vi "Data.vi"(11 "Message Queues out":T1) -> ()   [LabVIEW 2024]
doc: "This vi used for Data Logging Loop and its process"
uses:
  Message Queue/All Message Queues.ctl
  Message Queue/Message Cluster.ctl
  controls/GlobalData.ctl
  Message Queue/Enqueue Message (Single).vi
  <vilib>/Utility/error.llb/Error Cluster From Error Code.vi
  <vilib>/ErrorRing/Error Ring.xnode
  Message Queue/Message Queue.lvlib
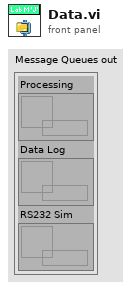
[diagram p1: front panel]
types:
  T1 = typedef "Message Queue.lvlib/All Message Queues.ctl" = cluster{"Processing":refnum<queue>, "Data Log":refnum<queue>, "RS232 Sim":refnum<queue>}
  T2 = typedef "GlobalData.ctl" = cluster{"Measurements":cluster{"Measurement Graphs":refnum<vi>, "Pressure":refnum<vi>, "Temperature":refnum<vi>, "Salinity":refnum<vi>, "Weight":refnum<vi>, "Pressure Raw":refnum<vi>, "Temperature Raw":refnum<vi>, "Salinity Raw":refnum<vi>, "Weight Raw":refnum<vi>, "Measurement Statstics":refnum<vi>, "Time Array":refnum<vi>}, "Settings":cluster{"Sampling Settings":refnum<vi>, "General Settings":refnum<vi>, "Disable Sensor Reading":refnum<vi>, "Units Settings":refnum<vi>, "Channels Settings":refnum<vi>, "Weight Port Settings":refnum<vi>}, "Calibration Data":cluster{"Pressure Cal":refnum<vi>, "Temperature Cal":refnum<vi>, "Salinity Cal":refnum<vi>, "Weight Cal":refnum<vi>}, "UI":cluster{"Generate Report":refnum<vi>}}
  T3 = enum16{"open", "open or create", "create or replace", "create", "open (read-only)"}
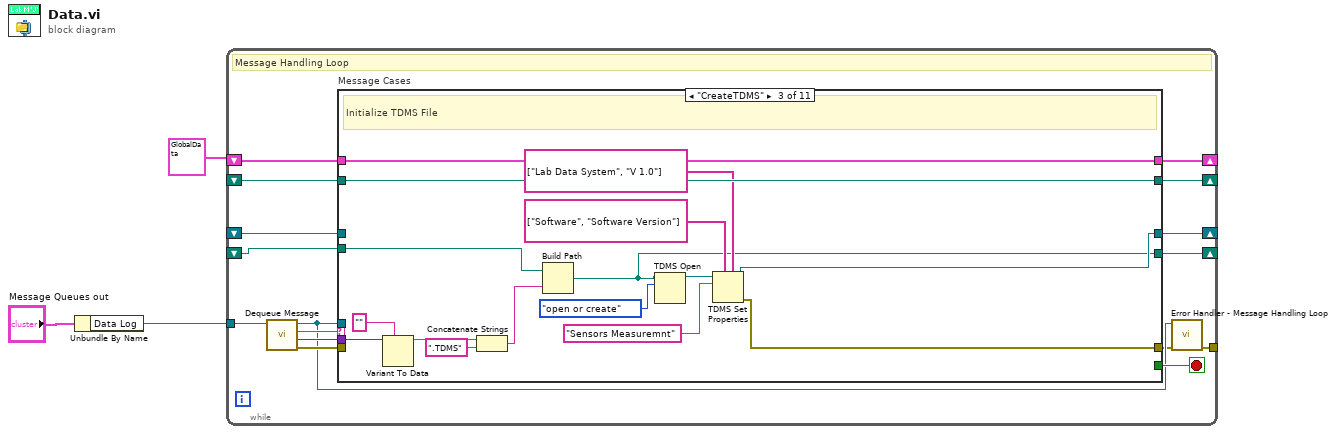
[diagram p0: block diagram]
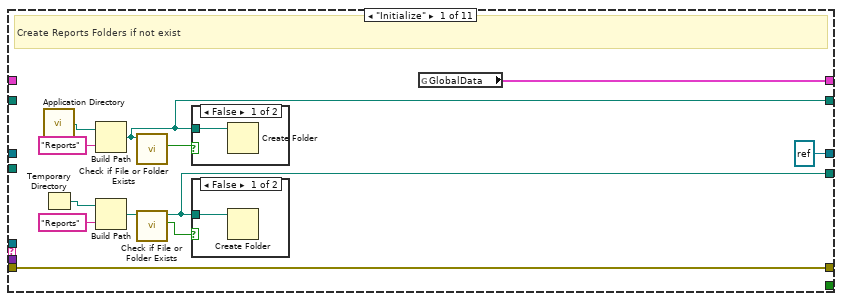
[diagram p2: hidden frame]
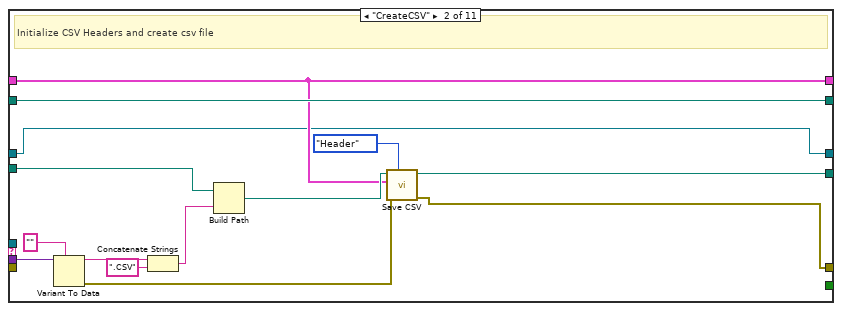
[diagram p5: hidden frame]
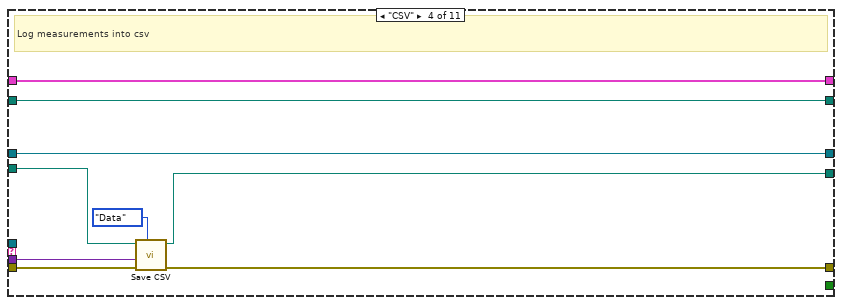
[diagram p6: hidden frame]
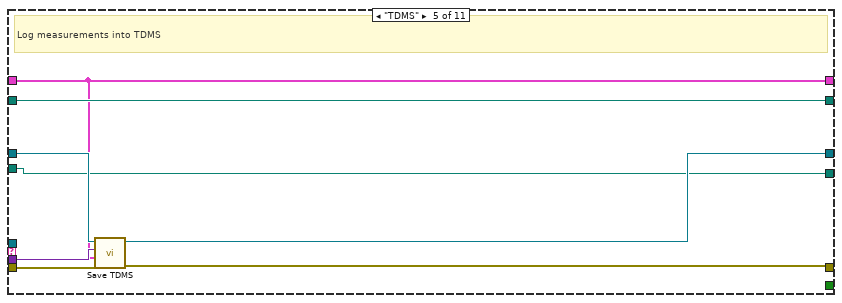
[diagram p7: hidden frame]
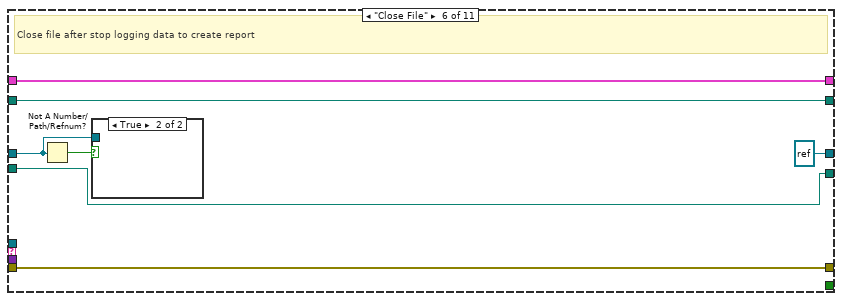
[diagram p8: hidden frame]
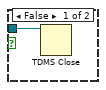
[diagram p9: hidden frame]
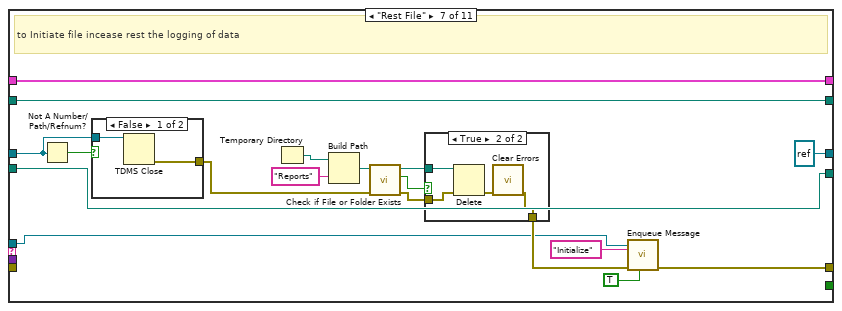
[diagram p10: hidden frame]
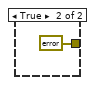
[diagram p12: hidden frame]
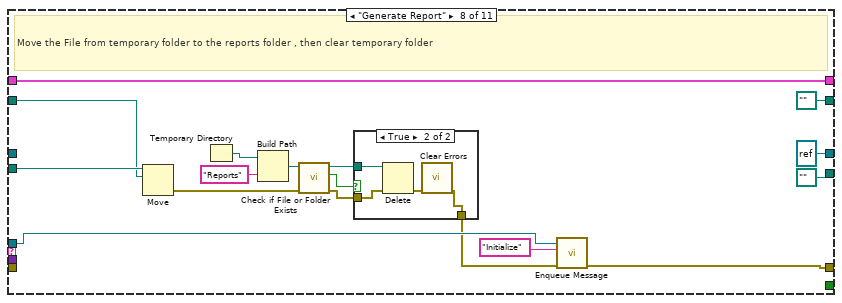
[diagram p13: hidden frame]
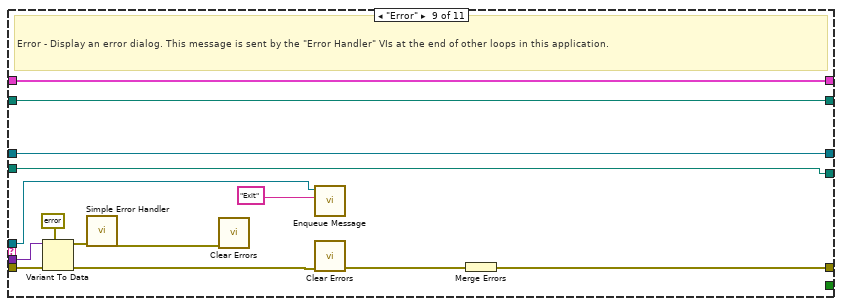
[diagram p15: hidden frame]
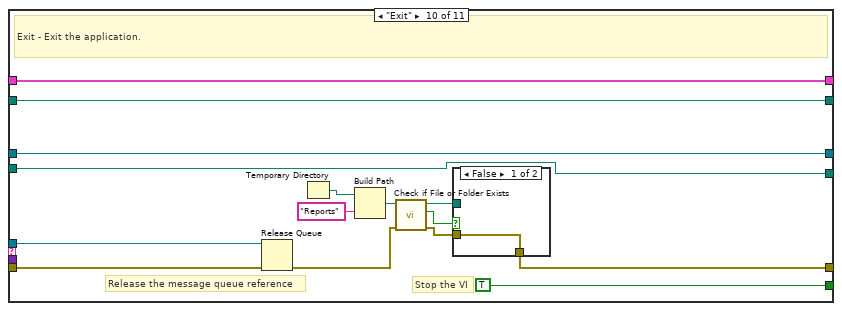
[diagram p16: hidden frame]
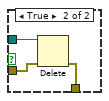
[diagram p17: hidden frame]
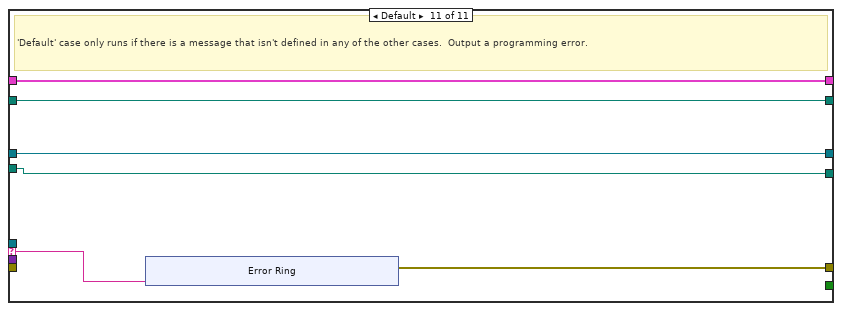
[diagram p18: hidden frame]
diagram:
  n1 = Unbundle By Name("Message Queues out") -> ("Data Log"=w3:refnum<queue>)
  n2 = while {
    shift-right: [w18] -> _
    shift-left: T2 {"Measurements"={"Measurement Graphs"=refnum, "Pressure"=refnum, "Temperature"=refnum, "Salinity"=refnum, "Weight"=refnum, "Pressure Raw"=refnum, "Temperature Raw"=refnum, "Salinity Raw"=refnum, "Weight Raw"=refnum, "Measurement Statstics"=refnum, "Time Array"=refnum}, "Settings"={"Sampling Settings"=refnum, "General Settings"=refnum, "Disable Sensor Reading"=refnum, "Units Settings"=refnum, "Channels Settings"=refnum, "Weight Port Settings"=refnum}, "Calibration Data"={"Pressure Cal"=refnum, "Temperature Cal"=refnum, "Salinity Cal"=refnum, "Weight Cal"=refnum}, "UI"={"Generate Report"=refnum}} ("GlobalData") -> [w19]
    tunnel: w3 -> [w4]
    tunnel: [w12] -> _
    shift-right: [w10] -> _
    shift-left: _ -> [w7]
    shift-right: [w9] -> _
    shift-left: _ -> [w8]
    shift-right: [w6] -> _
    shift-left: _ -> [w5]
    stop <- w17 stop-if-true
    # "Message Handling Loop"
    n3 = call "Dequeue Message.vi"("Message Queue"=w4) -> ("error out"=w16:errorcluster, "Message Data"=w14:variant, "Message"=w15:string, "dup Message Queue"=w13:refnum<queue>)  [unwired: 7 in]
    n4 = case "Message Cases" shown="\"CreateTDMS\"" w15 {
      selector: w15 -> [_ _ _ _ _ _ _ _ _ _ w173]
      tunnel: w13 -> [_ _ _ _ _ _ w91 w126 w137 w165 _]
      tunnel: w16 -> [w31 _ _ w69 w79 w87 _ _ w150 w162 _]
      tunnel: [w31 w35 w48 w66 w78 w87 w92 w127 w145 w155 w174] -> w11
      tunnel: w19 -> [_ w37 w63 w72 w73 w86 w106 w131 w149 w164 w175]
      tunnel: [w30 w37 w63 w72 w73 w86 w106 w131 w149 w164 w175] -> w18
      tunnel: [_ _ _ _ _ _ _ _ _ TRUE _] -> w17
      tunnel: w14 -> [_ w47 w62 w68 w76 _ _ _ w148 _ _]
      tunnel: [w22 w42 w56 w71 w74 w83 w103 path "" ("appended path") w144 w153 w170] -> w10
      tunnel: [w21 w40 w49 w65 w75 w81 w101 path "" ("new file path (Not A Path if cancelled)") w142 w151 w172] -> w9
      tunnel: w8 -> [_ w41 w57 w67 w75 w81 w101 w130 w142 w151 w172]
      tunnel: w7 -> [_ w42 w56 w71 w74 w83 w103 w129 w144 w153 w170]
      tunnel: [refnum<k34> refnum ("tdms file out") w34 w50 w70 w77 refnum<k34> refnum ("tdms file out") refnum<k34> refnum ("tdms file out") refnum<k34> refnum ("tdms file out") w143 w152 w171] -> w6
      tunnel: w5 -> [_ w34 _ w70 w80 w84 w104 _ w143 w152 w171]
      frame "Initialize" {
        # "Create Reports Folders if not exist"
        n5 = call <vilib>:"Application Directory.vi"() -> ("Application Directory"=w28:path)
        n6 = Temporary Directory() -> (w25:path)
        n7 = Build Path(base path=w28, name or relative path="Reports") -> (appended path=w22:path)
        n8 = Build Path(base path=w25, name or relative path="Reports") -> (appended path=w26:path)
        n9 = call <vilib>:"Check if File or Folder Exists.vi"("path"=w22) -> ("file or folder exists?"=w27:bool)  [unwired: 8 in, 2 out]
        n10 = call <vilib>:"Check if File or Folder Exists.vi"("path"=w26) -> ("file or folder exists?"=w23:bool, "dup path"=w21:path)  [unwired: 8 in, 1 out]
        n11 = case shown="False" w27 {
          tunnel: w22 -> [w33 _]
          frame False {
            n12 = Create Folder(path (use dialog)=w33) -> ()  [unwired: 2 in, 3 out]
          }
          frame True {
          }
        }
        n13 = case shown="False" w23 {
          tunnel: w21 -> [w32 _]
          frame False {
            n14 = Create Folder(path (use dialog)=w32) -> ()  [unwired: 2 in, 3 out]
          }
          frame True {
          }
        }
        n15 = global read "GlobalData.vi" "GlobalData"() -> (w30:T2)
      }
      frame "CreateCSV" {
        # "Initialize CSV Headers and create csv file"
        n16 = Variant To Data(type="", Variant=w47) -> (data=w45:string, error out=w36:errorcluster)  [unwired: 1 in]
        n17 = Concatenate Strings(w45, ".CSV" ("string")) -> (w43:string)
        n18 = Build Path(base path=w41, name or relative path=w43) -> (appended path=w39:path)
        n19 = call "Save CSV.vi"("CSV Type"=enum16{"Header", "Data"}."Header", "error in (no error)"=w36, "GlobalData"=w37, "file path (dialog if empty)"=w39) -> ("error out"=w35:errorcluster, "new file path (Not A Path if cancelled)"=w40:path)  [unwired: 6 in]
      }
      frame "CreateTDMS" {
        # "Initialize TDMS File"
        n20 = Variant To Data(type="", Variant=w62) -> (data=w60:string)  [unwired: 1 in, 1 out]
        n21 = Concatenate Strings(w60, ".TDMS" ("string")) -> (w58:string)
        n22 = Build Path(base path=w57, name or relative path=w58) -> (appended path=w49:path)
        n23 = TDMS Open(10:T3."open or create" ("operation (0:open)"), 11:w49) -> (3:w54:refnum<k34>)  [unwired: 5 in, 1 out]
        n24 = TDMS Set Properties(5:string[] ["Lab Data System", "V 1.0"] ("property names"), 7:string[] ["Software", "Software Version"] ("property names"), 10:"Sensors Measuremnt" ("group name"), 11:w54) -> (0:w48:errorcluster, 3:w50:refnum<k34>)  [unwired: 2 in, 2 out]
      }
      frame "CSV" {
        # "Log measurements into csv"
        n25 = call "Save CSV.vi"("CSV Type"=enum16{"Header", "Data"}."Data", "error in (no error)"=w69, "Data"=w68, "file path (dialog if empty)"=w67) -> ("error out"=w66:errorcluster, "new file path (Not A Path if cancelled)"=w65:path)  [unwired: 6 in]
      }
      frame "TDMS" {
        # "Log measurements into TDMS"
        n26 = call "Save TDMS.vi"("error in (no error)"=w79, "GlobalData"=w73, "Data"=w76, "tdms file in"=w80) -> ("error out"=w78:errorcluster, "tdms file out"=w77:refnum<k34>)  [unwired: 6 in]
      }
      frame "Close File" {
        # "Close file after stop logging data to create report"
        n27 = Not A Number/Path/Refnum?(number/path/refnum=w84) -> (NaN/Path/Refnum?=w85:bool)
        n28 = case shown="True" w85 {
          tunnel: w84 -> [w88 _]
          frame False {
            n29 = TDMS Close(11:w88) -> ()  [unwired: 1 in, 2 out]
          }
          frame True {
          }
        }
      }
      frame "Rest File" {
        # "to Initiate file incease rest the logging of data"
        n30 = Not A Number/Path/Refnum?(number/path/refnum=w104) -> (NaN/Path/Refnum?=w105:bool)
        n31 = case shown="False" w105 {
          tunnel: w104 -> [w113 _]
          tunnel: [w112 errorcluster {"status"=FALSE, "code"=0, "source"=""} ("error out")] -> w90
          frame False {
            n32 = TDMS Close(11:w113) -> (0:w112:errorcluster)  [unwired: 1 in, 1 out]
          }
          frame True {
          }
        }
        n33 = Temporary Directory() -> (w99:path)
        n34 = Build Path(base path=w99, name or relative path="Reports") -> (appended path=w100:path)
        n35 = call <vilib>:"Check if File or Folder Exists.vi"("error in (no error)"=w90, "path"=w100) -> ("error out"=w96:errorcluster, "file or folder exists?"=w98:bool, "dup path"=w97:path)  [unwired: 7 in]
        n36 = case shown="True" w98 {
          tunnel: w97 -> [_ w111]
          tunnel: w96 -> [w107 w110]
          tunnel: [w107 w108] -> w95
          frame False {
          }
          frame True {
            n37 = Delete(path (use dialog)=w111, error in=w110) -> (error out=w109:errorcluster)  [unwired: 3 in, 2 out]
            n38 = call <vilib>:"Clear Errors.vi"("error in (no error)"=w109) -> ("error out"=w108:errorcluster)  [unwired: 5 in, 1 out]
          }
        }
        n39 = call-poly "Enqueue Message.vi"("Priority Message? (F)"=TRUE, "error in (no error)"=w95, "Message"="Initialize", "Message Queue"=w91) -> ("error out"=w92:errorcluster)  [unwired: 6 in, 1 out]
      }
      frame "Generate Report" {
        # "Move the File from temporary folder to the reports folder , then clear temporary folder"
        n40 = Move(source path=w130, 10:w129) -> (error out=w119:errorcluster)  [unwired: 3 in, 2 out]
        n41 = Temporary Directory() -> (w124:path)
        n42 = Build Path(base path=w124, name or relative path="Reports") -> (appended path=w125:path)
        n43 = call <vilib>:"Check if File or Folder Exists.vi"("error in (no error)"=w119, "path"=w125) -> ("error out"=w120:errorcluster, "file or folder exists?"=w122:bool, "dup path"=w121:path)  [unwired: 7 in]
        n44 = case shown="True" w122 {
          tunnel: w121 -> [_ w136]
          tunnel: w120 -> [w132 w135]
          tunnel: [w132 w133] -> w118
          frame False {
          }
          frame True {
            n45 = Delete(path (use dialog)=w136, error in=w135) -> (error out=w134:errorcluster)  [unwired: 3 in, 2 out]
            n46 = call <vilib>:"Clear Errors.vi"("error in (no error)"=w134) -> ("error out"=w133:errorcluster)  [unwired: 5 in, 1 out]
          }
        }
        n47 = call-poly "Enqueue Message.vi"("error in (no error)"=w118, "Message"="Initialize", "Message Queue"=w126) -> ("error out"=w127:errorcluster)  [unwired: 7 in, 1 out]
      }
      frame "Error" {
        # "Error - Display an error dialog. This message is sent by the \"Error Handler\" VIs at the end of other loops in this application."
        n48 = Variant To Data(error in=w150, type=errorcluster {"status"=FALSE, "code"=0, "source"=""} ("error constant"), Variant=w148) -> (data=w146:errorcluster, error out=w140:errorcluster)
        n49 = call <vilib>:"Simple Error Handler.vi"("error in (no error)"=w146) -> ("error out"=w139:errorcluster)  [unwired: 4 in, 4 out]
        n50 = call <vilib>:"Clear Errors.vi"("error in (no error)"=w139) -> ()  [unwired: 5 in, 2 out]
        n51 = call-poly "Enqueue Message.vi"("Message"="Exit", "Message Queue"=w137) -> ()  [unwired: 8 in, 2 out]
        n52 = call <vilib>:"Clear Errors.vi"("error in (no error)"=w140) -> ("error out"=w141:errorcluster)  [unwired: 5 in, 1 out]
        n53 = Merge Errors(w141) -> (w145:errorcluster)
      }
      frame "Exit" {
        # "Stop the VI"
        # "Release the message queue reference"
        # "Exit - Exit the application."
        n54 = Release Queue(queue=w165, error in (no error)=w162) -> (error out=w154:errorcluster)  [unwired: 1 in, 2 out]
        n55 = Temporary Directory() -> (w160:path)
        n56 = Build Path(base path=w160, name or relative path="Reports") -> (appended path=w161:path)
        n57 = call <vilib>:"Check if File or Folder Exists.vi"("error in (no error)"=w154, "path"=w161) -> ("error out"=w156:errorcluster, "file or folder exists?"=w158:bool, "dup path"=w157:path)  [unwired: 7 in]
        n58 = case shown="False" w158 {
          tunnel: w157 -> [_ w169]
          tunnel: w156 -> [w166 w168]
          tunnel: [w166 w167] -> w155
          frame False {
          }
          frame True {
            n59 = Delete(path (use dialog)=w169, error in=w168) -> (error out=w167:errorcluster)  [unwired: 3 in, 2 out]
          }
        }
      }
      frame Default {
        # "'Default' case only runs if there is a message that isn't defined in any of the other cases.  Output a programming error."
        n60 = xnode "Error Ring"("parameter 0"=w173) -> ("error out"=w174:errorcluster)
      }
    }
    n61 = call "Error Handler - Message Handling Loop.vi"("error in (no error)"=w11, "Message Queue"=w13) -> ("dup error in"=w12:errorcluster)  [unwired: 8 in, 1 out]
  }
